vi "NGTS_ - Register PID Tags Sets RWs with SmartVIG .vi"(8 "error in":errorcluster, 11 "PID Tag Sets In":T1[](array[typedef])) -> (0 "error out":errorcluster, 3 "PID Tag Sets Out":T1[](array[typedef]))   [LabVIEW 2010]
doc: "This VI filters a system Tag list into sets of PID parameters and Gain Scheduling sets for each PID loop. It checks to see that each PID has all the correct parameters and that each Gain set has the correct number of parameters.\n\nThe standard PID input tag set is (example is loop# 001):\n\nPID_001_SP Setpoint\nPID_001_PV Process Variable\nPID_001_SPMAX Setpoint Max\nPID_001_SPMIN Setpoint Min\nPID_001_GSV Gain Schedule Variable\nPID_001_OUTH Output High Limit\nPID_001_OUTL Output Low Limit\nPID_001_MODE Mode: Auto (T) || Manaual (F)\nPID_001_MAN Value out in Manual Mode\n\nPlus at least one Gain Schedule Set of:\nPID_001_Pm Proportional\nPID_001_Im Integral\nPID_001_Dm Derivative\nPID_001_GSVMm GSVMax\n\nWhere m is the Gain Set number. The GSV is thresholded against the set of GSVMs to determine which Gain Set to use on a given loop iteration.\n\n2008_01_09 Mike Ashe\nmichael.ashe@imaginatics.net\nCell: 860-961-0876"
uses:
  Controls/NGTS_PID Loop Tag and Gain Set.ctl
  SmartBuffer_DBL/Public TypeDefs/SB_Operation Method.ctl
  SmartBuffer_DBL/SmartBuffer_DBL.lvlib
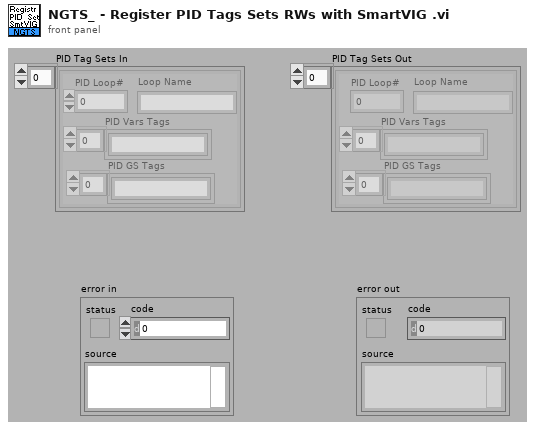
[diagram p1: front panel]
types:
  T1 = typedef "NGTS_PID Loop Tag and Gain Set.ctl" = cluster{"PID Loop#":i32, "PID Vars Tags":string[], "PID GS Tags":string[], "Loop Name":string}
  T2 = typedef "SmartBuffer_DBL.lvlib/SB_Operation Method.ctl" = enum16{"initialize", "register read op", "read data", "read data by tags", "register write op", "write data", "write data by tags", "import buffer image", "export buffer image", "register/replace read op", "register/replace write op"}
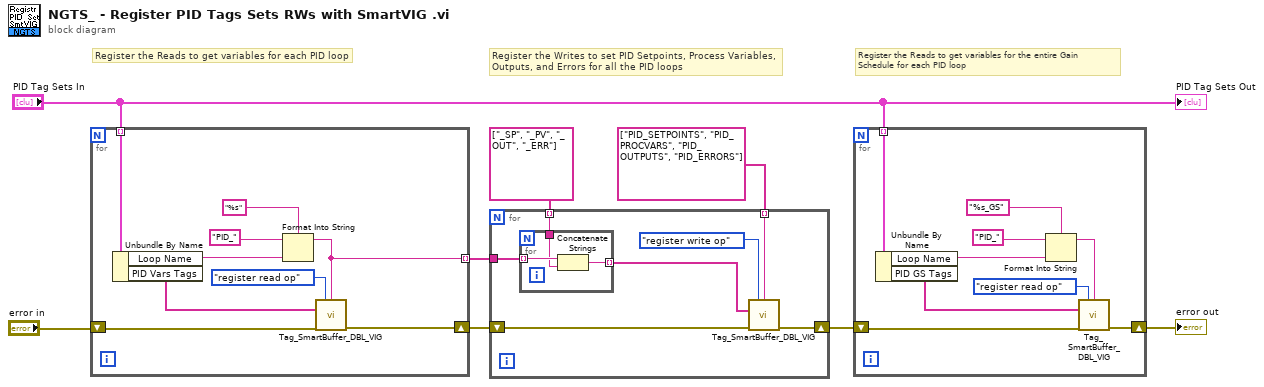
[diagram p0: block diagram]
diagram:
  # "Register the Writes to set PID Setpoints, Process Variables, \nOutputs, and Errors for all the PID loops"
  # "Register the Reads to get variables for the entire Gain\nSchedule for each PID loop"
  # "Register the Reads to get variables for each PID loop"
  n1 = for {
    tunnel: "PID Tag Sets In" -> [w16] mode=indexing
    shift-right: [w11] -> w6
    shift-left: "error in" -> [w12]
    tunnel: [w10] -> w2 mode=indexing
    n2 = Unbundle By Name(w16) -> ("Loop Name"=w15:string, "PID Vars Tags"=w13:string[])
    n3 = Format Into String(format string="%s", initial string="PID_" ("TagOp_Name"), w15) -> (resulting string=w10:string)  [unwired: 1 in, 1 out]
    n4 = call "Tag_SmartBuffer_DBL_VIG.vi"("SmartBuffer_Method"=SB_Operation_Method."register read op", "TagOp_Name"=w10, "tag_names_in"=w13, "error in"=w12) -> ("error out"=w11:errorcluster)  [unwired: 5 in, 6 out]
  }
  n5 = for {
    shift-right: [w23] -> w4
    shift-left: w6 -> [w24]
    tunnel: string[] ["_SP", "_PV", "_OUT", "_ERR"] -> [w20] mode=indexing
    tunnel: w2 -> [w21]
    tunnel: string[] ["PID_SETPOINTS", "PID_PROCVARS", "PID_OUTPUTS", "PID_ERRORS"] -> [w22] mode=indexing
    n6 = for {
      tunnel: w21 -> [w27] mode=indexing
      tunnel: w20 -> [w26]
      tunnel: [w25] -> w19 mode=indexing
      n7 = Concatenate Strings(w27, w26) -> (w25:string)
    }
    n8 = call "Tag_SmartBuffer_DBL_VIG.vi"("SmartBuffer_Method"=SB_Operation_Method."register write op", "TagOp_Name"=w22, "tag_names_in"=w19, "error in"=w24) -> ("error out"=w23:errorcluster)  [unwired: 5 in, 6 out]
  }
  n9 = for {
    tunnel: "PID Tag Sets In" -> [w34] mode=indexing
    shift-right: [w29] -> w7
    shift-left: w4 -> [w30]
    n10 = Unbundle By Name(w34) -> ("Loop Name"=w33:string, "PID GS Tags"=w31:string[])
    n11 = Format Into String(format string="%s_GS", initial string="PID_" ("TagOp_Name"), w33) -> (resulting string=w35:string)  [unwired: 1 in, 1 out]
    n12 = call "Tag_SmartBuffer_DBL_VIG.vi"("SmartBuffer_Method"=SB_Operation_Method."register read op", "TagOp_Name"=w35, "tag_names_in"=w31, "error in"=w30) -> ("error out"=w29:errorcluster)  [unwired: 5 in, 6 out]
  }
  "error out" <- w7
  "PID Tag Sets Out" <- "PID Tag Sets In"
